vi "Transfer ID to Tree Items.vi"(8 "error in (no error)":errorcluster, 9 "Transfer ID":string, 11 "Application Data in":T2) -> (0 "error out":errorcluster, 1 "Settings":T1, 2 "Item":T1, 3 "Application Data out":T2)   [LabVIEW 2017, in "DSF Mini Explorer.lvlib"]
uses:
  DSF Mini Explorer.lvlib
  Main VI/Application Data.ctl
  VeriStand/Data Sharing Custom Device/Source/DSF Core.lvlibp/Classes/Configuration/Configuration Session.lvclass
  Main VI/View Mode.ctl
  Tree Item.ctl
  Tree Item Type.ctl
  VeriStand/Data Sharing Custom Device/Source/DSF Core.lvlibp/Classes/Configuration/Read Settings.vi
  VeriStand/Data Sharing Custom Device/Source/DSF Core.lvlibp/Classes/Configuration/Read Transfer.vi
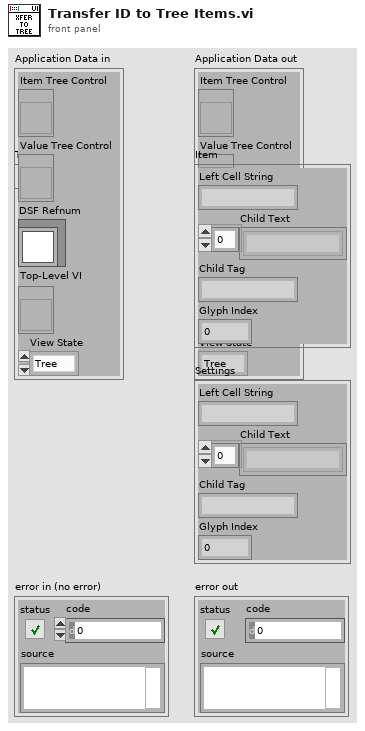
[diagram p1: front panel]
types:
  T1 = typedef "DSF Mini Explorer.lvlib/Tree Item.ctl" = cluster{"Left Cell String":string, "Child Text":string[], "Child Tag":string, "Glyph Index":i32}
  T2 = typedef "DSF Mini Explorer.lvlib/Application Data.ctl" = cluster{"Item Tree Control":refnum<vi>, "Value Tree Control":refnum<vi>, "DSF Refnum":refnum<class "Configuration Session.lvclass">, "Top-Level VI":refnum<vi>, "View State":T3}
  T3 = typedef "DSF Mini Explorer.lvlib/View Mode.ctl" = enum16{"Tree", "List"}
  T4 = typedef "DSF Mini Explorer.lvlib/Tree Item Type.ctl" = enum16{"Plugin", "Group", "Transfer", "Channel", "Setting"}
  T5 = typedef "DSF Core.lvlibp/DSF Transfer Info.ctl" = cluster{"byte order":T6, "channel ids":string[], "settings id":string}
  T6 = typedef "DSF Core.lvlibp/DSF Byte Order.ctl" = enum8{"big-endian", "little-endian"}
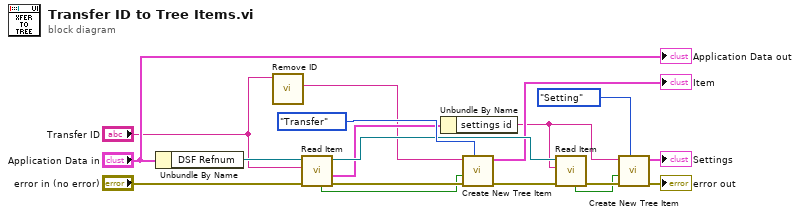
[diagram p0: block diagram]
diagram:
  n1 = Unbundle By Name("Application Data in") -> ("DSF Refnum"=w9:refnum<class "Configuration Session.lvclass">)
  n2 = call "Remove ID.vi"("id string"="Transfer ID") -> ("name"=w2:string)  [unwired: 8 in, 2 out]
  n3 = call-poly "Read Item.vi"("error in (no error)"="error in (no error)", "Transfer ID"="Transfer ID", "Configuration Session in"=w9) -> ("error out"=w14:errorcluster, "value"=w11:T5, "Configuration Session out"=w12:refnum<class "Configuration Session.lvclass">, "found?"=w4:bool)  [unwired: 5 in]
  n4 = Unbundle By Name(w11) -> ("settings id"=w1:string)
  n5 = call "Create New Tree Item.vi"("Item Type"=Tree_Item_Type."Transfer", "error in"=w14, "found?"=w4, "Left Cell String"=w2) -> ("error out"=w15:errorcluster, "Item"=→"Item":T1)  [unwired: 6 in]
  n6 = call-poly "Read Item.vi"("error in (no error)"=w15, "Settings ID"=w1, "Configuration Session in"=w12) -> ("error out"=w16:errorcluster, "found?"=w5:bool)  [unwired: 5 in, 2 out]
  n7 = call "Create New Tree Item.vi"("Item Type"=Tree_Item_Type."Setting", "error in"=w16, "found?"=w5, "Left Cell String"=w1) -> ("error out"=→"error out":errorcluster, "Item"=→"Settings":T1)  [unwired: 6 in]
  "Application Data out" <- "Application Data in"
